vi "Read (1 Parameter).vi"(8 "error in (no error)":errorcluster, 10 "Parameter (1: X)":u16(ring)=1 items=["X"=1, "Y"=2, "R"=3, "Theta"=4, "Channel 1"=5, "Channel 2"=6, "Aux In 1"=7, "Aux In 2"=8, "Aux In 3"=9, "Aux In 4"=10], 11 "VISA resource name":refnum<visa-resource-name>) -> (0 "error out":errorcluster, 2 "Measurement":dbl, 3 "VISA resource name out":refnum<visa-resource-name>)   [LabVIEW 2022 SP3, in "Stanford Research 830.lvlib"]
doc: "Reads single parameter and returns single measurement from the instrument."
uses:
  <instrlib>/Stanford Research 830/Stanford Research 830.lvlib
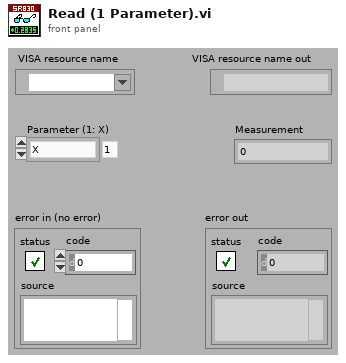
[diagram p1: front panel]
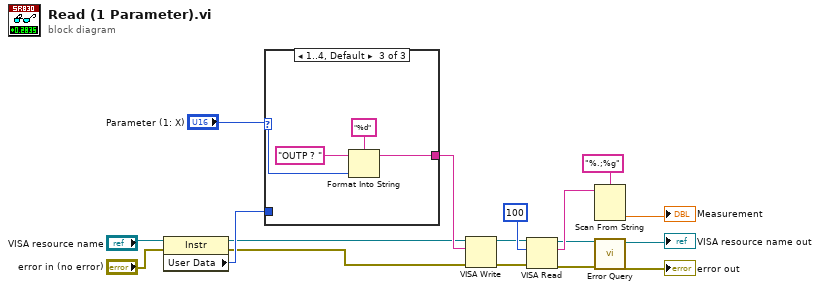
[diagram p0: block diagram]
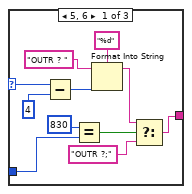
[diagram p2: hidden frame]
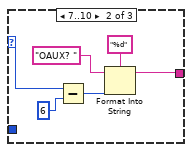
[diagram p3: hidden frame]
diagram:
  n1 = property class="Instr"(reference="VISA resource name", error in="error in (no error)") -> (reference out=w4:refnum<visa-resource-name>, error out=w3:errorcluster, "User Data"=w5:u32)
  n2 = case shown="1..4, Default" "Parameter (1: X)" {
    selector: "Parameter (1: X)" -> [w28 w30 w38]
    tunnel: [w18 w29 w35] -> w13
    tunnel: w5 -> [w23 _ _]
    frame 5, 6 {
      n3 = Subtract(x=w28, y=u16 4) -> (x-y=w26:u16)
      n4 = Equal?(x=u32 830, y=w23) -> (x = y?=w20:bool)
      n5 = Format Into String(format string="%d", initial string="OUTR ? ", w26) -> (resulting string=w21:string)  [unwired: 1 in, 1 out]
      n6 = Select(t=w21, s=w20, f="OUTR ?;") -> (s? t:f=w18:string)
    }
    frame 7..10 {
      n7 = Subtract(x=w30, y=u16 6) -> (x-y=w33:u16)
      n8 = Format Into String(format string="%d", initial string="OAUX? ", w33) -> (resulting string=w29:string)  [unwired: 1 in, 1 out]
    }
    frame 1..4, Default {
      n9 = Format Into String(format string="%d", initial string="OUTP ? " ("string (\"\")"), w38) -> (resulting string=w35:string)  [unwired: 1 in, 1 out]
    }
  }
  n10 = VISA Write(VISA resource name=w4, write buffer=w13, error in (no error)=w3) -> (VISA resource name out=w2:refnum<visa-resource-name>, error out=w1:errorcluster)  [unwired: 1 out]
  n11 = VISA Read(VISA resource name=w2, byte count=u32 100, error in (no error)=w1) -> (VISA resource name out=w9:refnum<visa-resource-name>, read buffer=w17:string, error out=w8:errorcluster)  [unwired: 1 out]
  n12 = Scan From String(format string="%.;%g", input string=w17) -> (output 1=→"Measurement":dbl)  [unwired: 3 in, 3 out]
  n13 = call <instrlib>:"Error Query.vi"("error in (no error)"=w8, "VISA resource name"=w9) -> ("error out"=→"error out":errorcluster, "VISA resource name out"=→"VISA resource name out":refnum<visa-resource-name>)  [unwired: 7 in, 1 out]
